vi "PolarizationRead.vi"(2 "error IO":errorcluster caption="error in") -> (0 "error IO 2":errorcluster caption="error out")   [LabVIEW 2018]
uses:
  <vilib>/Analysis/baseanly.llb/Mean (DBL).vi
  InOut/Reslut.vi
  <vilib>/Analysis/NI_AALBase.lvlib
panel:
  out "数组":dbl[](array[numeric])
  out "x+y":dbl
  out "偏振方向":dbl format="%0.2f"
  out "偏振度":dbl format="%0.2f"
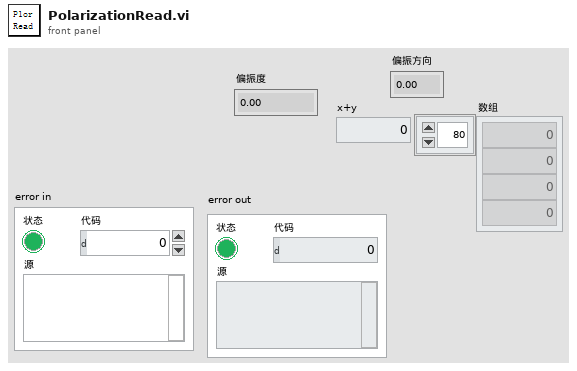
[diagram p1: front panel]
types:
  T1 = typedef "衰减片电机指令枚举器.ctl" = enum16{"归0", "停止", "运动", "轴设置", "通信连接"}
  T2 = typedef "衰减片电机枚举.ctl" = enum16{"小积分球衰减", "偏振仪衰减", "近场相机衰减", "远场相机衰减"}
  T3 = typedef "控制电机位置枚举器.ctl" = enum16{"远场扫描", "发散角扫描", "远场相机", "近场相机", "时间波形", "偏振", "能量", "功率", "光谱"}
  T4 = typedef "控制电机指令枚举器.ctl" = enum16{"归0", "停止", "运动", "轴设置", "通信连接"}
  T5 = typedef "控制电机枚举器.ctl" = enum16{"Z", "Y", "X", "发散角", "俯仰", "旋转"}
  T6 = typedef "衰减片电机位置枚举器.ctl" = enum16{"0倍", "10倍", "100倍", "1000倍"}
  T7 = cluster{"激光器型号":string, "X":dbl, "Y":dbl, "Z":dbl, "Rotate":dbl, "Pitching":dbl, "DivergeAngle":dbl, "衰减片位置":cluster{"小积分球位置":T6, "偏振仪位置 ":T6, "近场相机位置 ":T6, "远场相机位置":T6}, "Type":string, "Serial":string}
  T8 = cluster{" 偏振方向":string, "偏振度":string, " 偏振方向 单位 ":string, "偏振度单位":string}
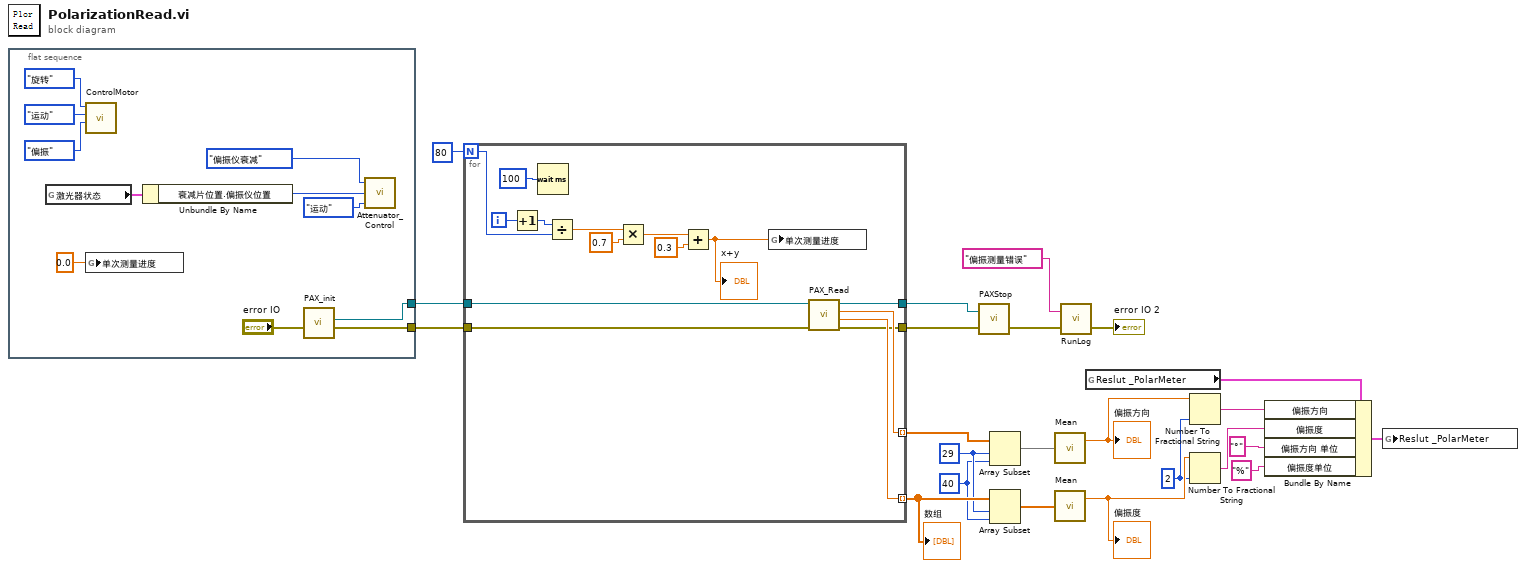
[diagram p0: block diagram]
diagram:
  w1 = 40 ("长度")
  w2 = 29 ("索引")
  w7 = i16 2 ("精度(6)")
  n1 = flat-sequence {
    tunnel: [w34] -> w12
    tunnel: [w33] -> w11
    frame #0 {
      n2 = global read "参数.vi" "激光器状态"() -> (w27:T7)
      n3 = call "ControlMotor.vi"("控制电机"=控制电机枚举器."旋转", "控制电机指令"=控制电机指令枚举器."运动", "位置"=控制电机位置枚举器."偏振") -> ()  [unwired: 5 in, 1 out]
      n4 = global write "globalMessage.vi" "单次测量进度"(0.0 ("单次测量进度")) -> ()
      n5 = Unbundle By Name(w27) -> ("衰减片位置.偏振仪位置"=w26:T6)
      n6 = call "PAX_init.vi"("Error In"="error IO") -> ("error out"=w33:errorcluster, "偏振测量仪VISA"=w34:refnum<visa-resource-name>)  [unwired: 9 in]
      n7 = call "Attenuator_Control.vi"("控制电机指令"=衰减片电机指令枚举器."运动", "位置"=w26, "电机"=衰减片电机枚举."偏振仪衰减") -> ()  [unwired: 2 in, 1 out]
    }
  }
  n8 = for {
    N: 80 -> [w41]
    tunnel: w11 -> [w48]
    tunnel: w12 -> [w49]
    tunnel: [w47] -> w6 mode=indexing
    tunnel: [w46] -> w4 mode=indexing
    tunnel: [w45] -> w9
    tunnel: [w44] -> w10
    i -> [w42]
    n9 = Increment(x=w42) -> (x+1=w35:i32)
    n10 = Wait (ms)(milliseconds to wait=u32 100 ("等待时间（毫秒）")) -> ()  [unwired: 1 out]
    n11 = Divide(x=w35, y=w41) -> (x/y=w36:dbl)
    n12 = Multiply(x=w36, y=0.7) -> (x*y=w40:dbl)
    n13 = Add(x=w40, y=0.3) -> (x+y=w38:dbl)
    "x+y" <- w38
    n14 = global write "globalMessage.vi" "单次测量进度"(w38) -> ()
    n15 = call "PAX_Read.vi"("error in (no error)"=w48, "VISA in"=w49) -> ("error out"=w45:errorcluster, "DOP"=w46:dbl, "Azimuth deg"=w47:dbl, "VISAout"=w44:refnum<visa-resource-name>)  [unwired: 2 in, 4 out]
  }
  "数组" <- w4
  n16 = call "PAXStop.vi"("error in"=w9, "VISA 输入"=w10) -> ("error out"=w8:errorcluster)  [unwired: 1 in]
  n17 = Array Subset(array=w6, index=w2, length=w1) -> (w5:dbl[])
  n18 = Array Subset(array=w4, index=w2, length=w1) -> (w3:dbl[])
  n19 = call-poly <vilib>:"Mean.vi"("X"=w5) -> ("mean"=w19:dbl)  [unwired: 1 out]
  "偏振方向" <- w19
  n20 = call-poly <vilib>:"Mean.vi"("X"=w3) -> ("mean"=w16:dbl)  [unwired: 1 out]
  "偏振度" <- w16
  n21 = call "RunLog.vi"("error in"=w8, "Message"="偏振测量错误") -> ("error out"=→"error IO 2":errorcluster)  [unwired: 1 in]
  n22 = global read "Reslut.vi" "Reslut _PolarMeter"() -> (w20:T8)
  n23 = Number To Fractional String(number=w19, precision (6)=w7) -> (F-format string=w18:string)  [unwired: 2 in]
  n24 = Number To Fractional String(number=w16, precision (6)=w7) -> (F-format string=w15:string)  [unwired: 2 in]
  n25 = Bundle By Name(cluster=w20, "偏振方向"=w18, "偏振度"=w15, "偏振方向 单位"="°" ("偏振度"), "偏振度单位"="%") -> (w13:T8)
  n26 = global write "Reslut.vi" "Reslut _PolarMeter"(w13) -> ()
